vi "Plant1.vi"(8 "error in (no error)":errorcluster) -> (0 "error out":errorcluster)   [LabVIEW 2016]
uses:
  <vilib>/Platform/TimedLoop/XDataNode/timing_clust.ctl
  <vilib>/Platform/TimedLoop/XDataNode/nitl_modes.ctl
  <vilib>/Platform/TimedLoop/XDataNode/wakeup.ctl
  <vilib>/Model Interface Toolkit/Model Interface Toolkit.lvclass/Model Interface Toolkit.ctl
  <vilib>/Model Interface Toolkit/Model Update.vi
  <vilib>/Model Interface Toolkit/Tick Model.vi
  <vilib>/Model Interface Toolkit/Probe Signals.vi
  <vilib>/Model Interface Toolkit/Multirate/Dispatch Model Tasks.vi
  <vilib>/Model Interface Toolkit/Call Model Start Routine.vi
  <vilib>/Model Interface Toolkit/Handle Error.vi
  <vilib>/Model Interface Toolkit/Multirate/Wait on Tasks.vi
  <vilib>/xnet/xnet.llb/XNET Read (Signal Single-point).vi
  <vilib>/Model Interface Toolkit/Check Error.vi
  <vilib>/Model Interface Toolkit/Generate Error Cluster.vi
  <vilib>/Platform/TimedLoop/scheduler/LVUserAPI/Fire Software-Triggered Timing Source.vi
  <vilib>/Platform/TimedLoop/XDataNode/XDataNode.xnode
  <vilib>/Platform/TimedLoop/XDataNode/XDNodeRunTimeDep.lvlib
  <vilib>/Model Interface Toolkit/Model Interface Toolkit.lvclass
panel:
  in  "stop":bool
  out "Model Period (s)":dbl=0.2
  out "Waveform Chart":cluster{dbl, dbl, dbl}(graph)
  out "Bus data":dbl[](array[numeric])
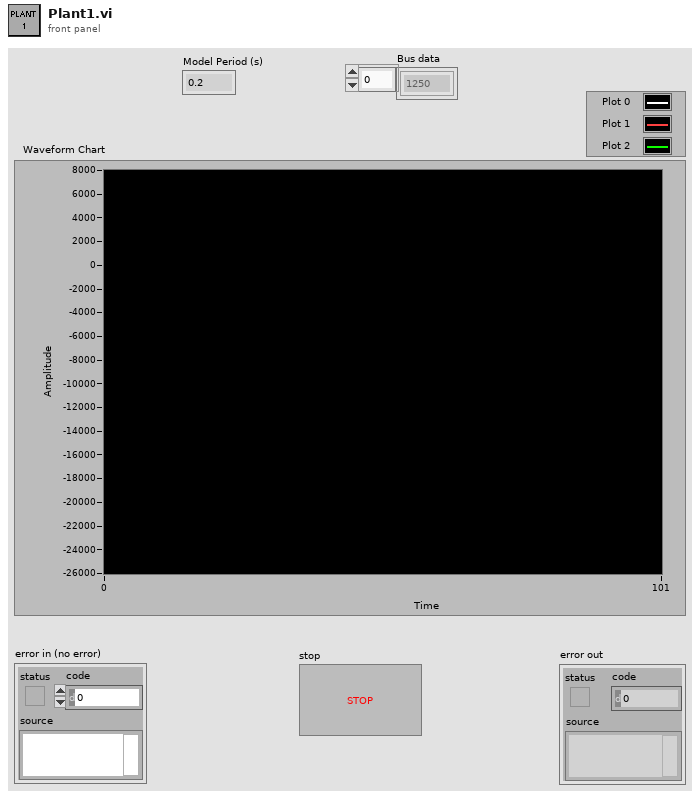
[diagram p1: front panel]
types:
  T1 = typedef "XDNodeRunTimeDep.lvlib/timing_clust.ctl" = cluster{"Expected End [f-1]":u64, "Actual End [f-1]":u64, "Finished Late? [f-1]":bool, "Expected End [i-1]":u64, "Actual End [i-1]":u64, "Finished Late? [i-1]":bool, "Expected Start [i]":u64, "Actual Start [i]":u64, "Expected Start [f]":u64, "Actual Start [f]":u64, "Source Name":string, "Structure Name":string, "Period":i64, "Deadline":i64, "Offset":i64, "Start":i64, "Priority":i32, "Timeout":i32, "Mode":T2, "Wakeup Reason":T3, "Error":errorcluster, "Source Type":string, "Secondary Source Type":string, "Global End Time":u64, "Global Start Time":u64, "Frame Duration":u64, "Iteration Duration":u64, "Assigned CPU":i32, "I/O Scan Engine Mode":u32}
  T2 = typedef "XDNodeRunTimeDep.lvlib/nitl_modes.ctl" = enum32{"No Change", "Process missed periods, maintain original phase", "Discard missed periods, maintain original phase", "Process missed periods, ignore original phase", "Discard missed periods, ignore original phase"}
  T3 = typedef "XDNodeRunTimeDep.lvlib/wakeup.ctl" = enum32{"Normal", "Aborted", "Asynchronous wakeup", "Timing source error", "Timed loop error", "Timeout"}
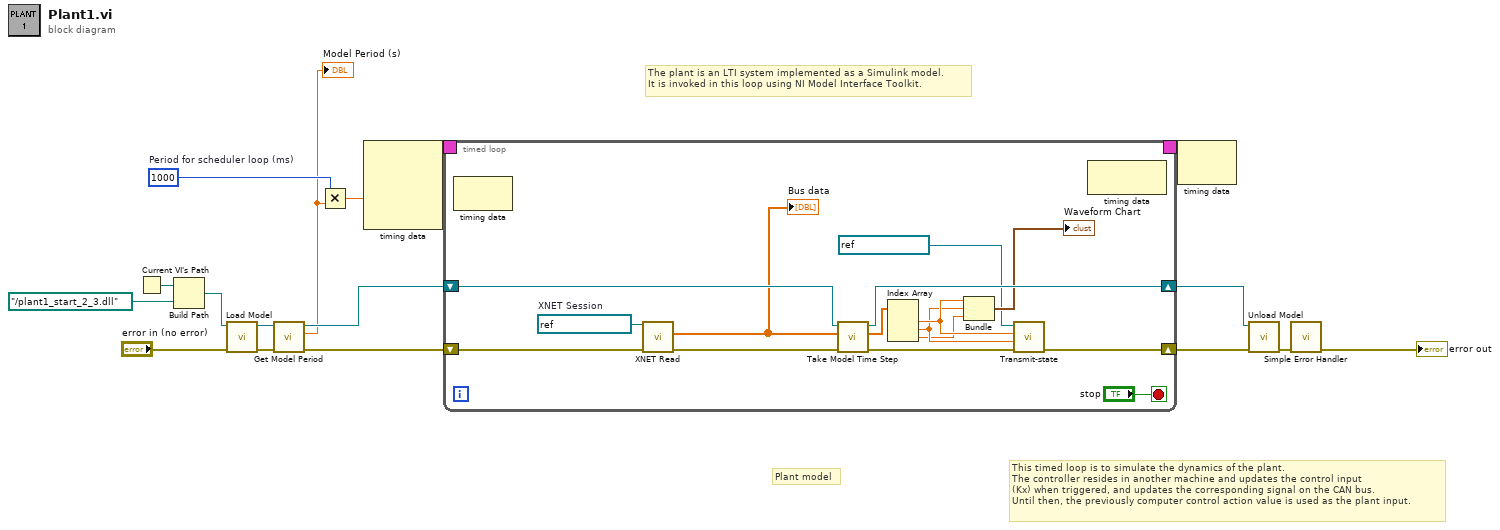
[diagram p0: block diagram]
diagram:
  w7 = i64 1000  # Period for scheduler loop (ms)
  # "Plant model"
  # "This timed loop is to simulate the dynamics of the plant.\nThe controller resides in another machine and updates the control input\n(Kx) when triggered, and updates the corresponding signal on the CAN bus. \nUntil then, the previously computer control action value is used as the plant input."
  # "The plant is an LTI system implemented as a Simulink model.\nIt is invoked in this loop using NI Model Interface Toolkit."
  n1 = Current VI's Path() -> (path=w12:path)
  n2 = Build Path(base path=w12, name or relative path=path "../plant1_start_2_3.dll" ("Model Path")) -> (appended path=w11:path)
  n3 = call <vilib>:"Load Model.vi"("error in (no error)"="error in (no error)", "Model Path"=w11) -> ("error out"=w14:errorcluster, "Model out"=w15:refnum<class "Model Interface Toolkit.lvclass">)  [unwired: 8 in]
  n4 = call <vilib>:"Get Model Period.vi"("error in"=w14, "Model in"=w15) -> ("error out"=w4:errorcluster, "Model Period (s)"=w6:dbl, "Model out"=w8:refnum<class "Model Interface Toolkit.lvclass">)  [unwired: 7 in]
  "Model Period (s)" <- w6
  n5 = Multiply(x=w7, y=w6) -> (x*y=w5:dbl)
  n6 = node-c288(w5) -> (w17:T1)  [unwired: 3 in]
  n7 = timed-loop {
    timing: w17 -> [_]
    timing-out: [_] -> w16
    shift-right: [w31] -> w2
    shift-left: w8 -> [w32]
    shift-right: [w27] -> w3
    shift-left: w4 -> [w23]
    stop <- "stop" stop-if-true
    w24 = refnum<k21> "Plant1_input"  # XNET Session
    n8 = node-c288() -> ()  [unwired: 1 in, 1 out]
    n9 = call-poly <vilib>:"XNET Read.vi"("session in"=w24, "error in (no error)"=w23) -> ("data"=w21:dbl[], "error out"=w22:errorcluster)  [unwired: 11 in, 1 out]
    "Bus data" <- w21
    n10 = call <vilib>:"Take Model Time Step.vi"("error in (no error)"=w22, "Inport Array"=w21, "Model in"=w32) -> ("error out"=w28:errorcluster, "Outport Array out"=w30:dbl[], "Model out"=w31:refnum<class "Model Interface Toolkit.lvclass">)  [unwired: 6 in]
    n11 = Index Array(array=w30) -> (element #1=w26:dbl, element #2=w25:dbl, element #3=w20:dbl)  [unwired: 3 in]
    n12 = Bundle(w26, w25, w20) -> (→"Waveform Chart":cluster{dbl, dbl, dbl})  [unwired: 1 in]
    n13 = call "Transmit-state.vi"("error in (no error)"=w28, "X2"=w25, "X1"=w26, "XNET Session"=refnum<k21> "Plant1_state") -> ("error out"=w27:errorcluster)  [unwired: 7 in]
    n14 = node-c288() -> ()  [unwired: 1 in, 1 out]
  }
  n15 = node-c288(w16) -> ()  [unwired: 1 out]
  n16 = call <vilib>:"Unload Model.vi"("error in (no error)"=w3, "Model in"=w2) -> ("error out"=w10:errorcluster)  [unwired: 9 in]
  n17 = call <vilib>:"Simple Error Handler.vi"("error in (no error)"=w10) -> ("error out"=→"error out":errorcluster)  [unwired: 4 in, 4 out]
